vi "System2.vi"() -> ()   [LabVIEW 2013]
uses:
  <vilib>/imath/engines/lvmath/Functions/Error Handling/error.ctl
  <vilib>/imath/engines/lvmath/Plug In/_Char/NIMS_CH_character datatype.ctl
  <instrlib>/niUSRP/niUSRP Fetch Rx Data (CDB).vi
  <vilib>/imath/engines/lvmath2/RunTimeEngine/ErrorHandling/NIMS_Finalize Error.vi
  <vilib>/imath/engines/lvmath2/RunTimeEngine/Managers/WorkSpace/UID Generator.vi
  <vilib>/imath/engines/lvmath2/RunTimeEngine/NonStaticBuiltInFunctions/Manual/NIMS_NS_load.vi
  <vilib>/imath/engines/lvmath2/RunTimeEngine/RunTimeType/NIMS_RunTimeType_From StrictType (excl LVString).vi
  <instcachedir>/0/NIMS_RunTimeType_From StrictType (excl LVString)_4DEE718D6EB74582AA20236969C084FC.lvgen/NIMS_RunTimeType_From StrictType (excl LVString)_4DEE718D6EB74582AA20236969C084FC_000.vi
  <vilib>/imath/engines/lvmath2/RunTimeEngine/Managers/SymbolTable/Write Variable.vi
  <vilib>/imath/engines/lvmath2/RunTimeEngine/RowToken/NIMS_RowToken-nonstatic.vi
  <vilib>/imath/engines/lvmath2/RunTimeEngine/MatrixToken/NIMS_MatrixToken-nonstatic.vi
  <vilib>/imath/engines/lvmath2/RunTimeEngine/RunTimeSymbolToken/NIMS_RunTimeSymbolToken_ReadVariable-1out.vi
  <vilib>/imath/engines/lvmath/Functions/Error Handling/MergeErrorsWrapper.vi
  <vilib>/imath/engines/lvmath2/RunTimeEngine/LocalVariableDefStatement/MC_LocalVariableDefStatement_Display.vi
  <vilib>/imath/engines/lvmath2/RunTimeEngine/RunTimeSymbolToken/NIMS_RunTimeSymbolToken_ResolveSymbol.vi
  <instcachedir>/0/NIMS_RunTimeSymbolToken_ResolveSymbol_F94DACEDB8D84373A3303A9E667D843C.lvgen/NIMS_RunTimeSymbolToken_ResolveSymbol_F94DACEDB8D84373A3303A9E667D843C_003.vi
  <vilib>/imath/engines/lvmath2/RunTimeEngine/CommandStatement/NIMS_CommandStatement_MaskErr.vi
  <vilib>/imath/engines/lvmath2/RunTimeEngine/Managers/SymbolTable/Read Variable.vi
  <vilib>/imath/engines/lvmath2/RunTimeEngine/RunTimeType/NIMS_RunTimeType_Get Case Value.vi
  <vilib>/imath/engines/lvmath2/RunTimeEngine/NodeEndStatement/MC_NodeEndStatement_Dispose.vi
  <vilib>/imath/engines/lvmath2/RunTimeEngine/NodeEndStatement/NIMS_NodeEndStatement_Output.vi
  <instcachedir>/0/NIMS_NodeEndStatement_Output_53EC0D466D134D7ABD903AC30B43404B.lvgen/NIMS_NodeEndStatement_Output_53EC0D466D134D7ABD903AC30B43404B_004.vi
  <vilib>/imathl/engines/lvmath/Functions/Error Handling/Create Error.vi
  <vilib>/imath/engines/lvmath2/RunTimeEngine/RunTimeType/NIMS_RunTimeType_To Numeric.vi
  <instcachedir>/0/NIMS_RunTimeType_To Numeric_4795FB10E831402FABFA341B47E20681.lvgen/NIMS_RunTimeType_To Numeric_4795FB10E831402FABFA341B47E20681_000.vi
  <vilib>/imath/engines/lvmath2/RunTimeEngine/NodeEndStatement/NIMS_NodeEndStatement_Get Vector.vi
  <instcachedir>/0/NIMS_NodeEndStatement_Get Vector_BE4364D373AE46158CA0B14DEB6F98C8.lvgen/NIMS_NodeEndStatement_Get Vector_BE4364D373AE46158CA0B14DEB6F98C8_003.vi
  <vilib>/imath/engines/lvmath/Plug In/_Char/RunTimeType/NIMS_CH_RunTimeType_To Character 2D.vi
  <instcachedir>/0/NIMS_NodeEndStatement_Get Vector_BE4364D373AE46158CA0B14DEB6F98C8.lvgen/NIMS_NodeEndStatement_Get Vector_BE4364D373AE46158CA0B14DEB6F98C8_000.vi
  <vilib>/imath/engines/lvmath/Plug In/_Char/NIMS_CH_Character 1D to U8 1D.vi
  <vilib>/imath/engines/lvmath2/RunTimeEngine/BuiltInFunctions/crosscorr/NIMS_crosscorr(GV,GV,Str).vi
  <instcachedir>/0/NIMS_crosscorr(GV,GV,Str)_7F516622EB1B4986A7D0F3F178AC2F2E.lvgen/NIMS_crosscorr(GV,GV,Str)_7F516622EB1B4986A7D0F3F178AC2F2E_000.vi
  <vilib>/imath/engines/lvmath2/RunTimeEngine/BuiltInFunctions/abs/NIMS_abs(signed).vi
  <instcachedir>/0/NIMS_abs(signed)_C4FCB8E6058B49B797C7C8D53CA5F6EC.lvgen/NIMS_abs(signed)_C4FCB8E6058B49B797C7C8D53CA5F6EC_006.vi
  <vilib>/imath/engines/lvmath2/RunTimeEngine/BuiltInFunctions/length/NIMS_length(GV).vi
  <instcachedir>/0/NIMS_length(GV)_08A3D13377FD4E4B96F5795FBF3698FA.lvgen/NIMS_length(GV)_08A3D13377FD4E4B96F5795FBF3698FA_001.vi
  <vilib>/imath/engines/lvmath2/RunTimeEngine/RangeToken/NIMS_Range_R2 - Integer.vi
  <instcachedir>/0/NIMS_Range_R2 - Integer_C51C130E5EA5464EA148B28CDAB9615A.lvgen/NIMS_Range_R2 - Integer_C51C130E5EA5464EA148B28CDAB9615A_000.vi
  <instcachedir>/0/NIMS_NodeEndStatement_Output_53EC0D466D134D7ABD903AC30B43404B.lvgen/NIMS_NodeEndStatement_Output_53EC0D466D134D7ABD903AC30B43404B_014.vi
  <instcachedir>/0/NIMS_NodeEndStatement_Output_53EC0D466D134D7ABD903AC30B43404B.lvgen/NIMS_NodeEndStatement_Output_53EC0D466D134D7ABD903AC30B43404B_011.vi
  <vilib>/imath/engines/lvmath2/RunTimeEngine/IndexRead/NIMS V(S).vi
  <instcachedir>/0/NIMS V(S)_0488751826AF41519A22953C041130DC.lvgen/NIMS V(S)_0488751826AF41519A22953C041130DC_005.vi
  <instcachedir>/0/NIMS_abs(signed)_C4FCB8E6058B49B797C7C8D53CA5F6EC.lvgen/NIMS_abs(signed)_C4FCB8E6058B49B797C7C8D53CA5F6EC_002.vi
  <vilib>/imath/engines/lvmath2/RunTimeEngine/ErrorHandling/NIMS_Create Error From Enums.vi
  <vilib>/imath/engines/lvmath2/RunTimeEngine/Managers/SymbolTable/Clear UID.vi
  <vilib>/imath/engines/lvmath2/RunTimeEngine/BuiltInFunctions/close/NIMS_close(Enums).vi
  <vilib>/imath/engines/lvmath2/RunTimeEngine/BuiltInFunctions/figure/NIMS_figure(I32).vi
  <vilib>/imath/engines/lvmath2/RunTimeEngine/BuiltInFunctions/plot/NIMS_plot(G, Str).vi
  <instcachedir>/0/NIMS_plot(G, Str)_30D49D8623E0484DBD39D394DDFCBE95.lvgen/NIMS_plot(G, Str)_30D49D8623E0484DBD39D394DDFCBE95_000.vi
  <instcachedir>/0/NIMS_NodeEndStatement_Output_53EC0D466D134D7ABD903AC30B43404B.lvgen/NIMS_NodeEndStatement_Output_53EC0D466D134D7ABD903AC30B43404B_000.vi
  <instcachedir>/0/NIMS_NodeEndStatement_Output_53EC0D466D134D7ABD903AC30B43404B.lvgen/NIMS_NodeEndStatement_Output_53EC0D466D134D7ABD903AC30B43404B_001.vi
  <vilib>/imath/engines/lvmath/Plug In/_Char/NIMS_CH_Character RV to String.vi
  <instcachedir>/0/NIMS_plot(G, Str)_30D49D8623E0484DBD39D394DDFCBE95.lvgen/NIMS_plot(G, Str)_30D49D8623E0484DBD39D394DDFCBE95_001.vi
  <vilib>/imath/engines/lvmath2/RunTimeEngine/BuiltInFunctions/hold/NIMS_hold(Enums).vi
  <vilib>/imath/engines/lvmath2/RunTimeEngine/IndexRead/NIMS V(R2).vi
  <instcachedir>/0/NIMS V(R2)_C76619605A0E4E9F8B2FA9389712AC47.lvgen/NIMS V(R2)_C76619605A0E4E9F8B2FA9389712AC47_001.vi
  <vilib>/imath/engines/lvmath2/RunTimeEngine/BuiltInFunctions/max/1 input/NIMS_max(RV).vi
  <instcachedir>/0/NIMS_max(RV)_237633DB1D604D5BA7001287DF3C7957.lvgen/NIMS_max(RV)_237633DB1D604D5BA7001287DF3C7957_000.vi
  <instcachedir>/0/NIMS_length(GV)_08A3D13377FD4E4B96F5795FBF3698FA.lvgen/NIMS_length(GV)_08A3D13377FD4E4B96F5795FBF3698FA_002.vi
  <vilib>/imath/engines/lvmath2/RunTimeEngine/BuiltInFunctions/angle/NIMS_angle.vi
  <instcachedir>/0/NIMS_angle_6DDAE2BD99E0421EB990B6436E94D88F.lvgen/NIMS_angle_6DDAE2BD99E0421EB990B6436E94D88F_005.vi
  <vilib>/imath/engines/lvmath2/RunTimeEngine/BuiltInFunctions/imag/NIMS_imag(Complex).vi
  <instcachedir>/0/NIMS_imag(Complex)_3180D40D00C843A49C2B33397F857BF3.lvgen/NIMS_imag(Complex)_3180D40D00C843A49C2B33397F857BF3_002.vi
  <vilib>/imath/engines/lvmath2/RunTimeEngine/RangeToken/NIMS_Range.vi
  <instcachedir>/0/NIMS_Range_7481B155BEE341ECA0F59DDB444E2C09.lvgen/NIMS_Range_7481B155BEE341ECA0F59DDB444E2C09_001.vi
  <vilib>/imath/engines/lvmath2/RunTimeEngine/IndexRead/NIMS V(V).vi
  <instcachedir>/0/NIMS V(V)_298D9CB7BFEB42B8BC8D9C3C28AE8C70.lvgen/NIMS V(V)_298D9CB7BFEB42B8BC8D9C3C28AE8C70_000.vi
  <vilib>/imath/engines/lvmath2/RunTimeEngine/BuiltInFunctions/mean/NIMS_CS=mean(CV,I32).vi
  <instcachedir>/0/NIMS_angle_6DDAE2BD99E0421EB990B6436E94D88F.lvgen/NIMS_angle_6DDAE2BD99E0421EB990B6436E94D88F_003.vi
  <vilib>/imath/engines/lvmath2/RunTimeEngine/BuiltInFunctions/mean/NIMS_RS=mean(RV,I32).vi
  <instcachedir>/0/NIMS_abs(signed)_C4FCB8E6058B49B797C7C8D53CA5F6EC.lvgen/NIMS_abs(signed)_C4FCB8E6058B49B797C7C8D53CA5F6EC_000.vi
  <vilib>/imath/engines/lvmath2/RunTimeEngine/BuiltInFunctions/linramp/NIMS_linramp.vi
  <vilib>/imath/engines/lvmath2/RunTimeEngine/ArithmeticOperatorToken/NIMS_ArithmeticOperator_plus.vi
  <instcachedir>/0/NIMS_ArithmeticOperator_plus_8A46DAFC24D445C9B2C97B626139369E.lvgen/NIMS_ArithmeticOperator_plus_8A46DAFC24D445C9B2C97B626139369E_005.vi
  <vilib>/imath/engines/lvmath2/RunTimeEngine/BuiltInFunctions/numelements/NIMS_numelements.vi
  <instcachedir>/0/NIMS_numelements_A776DA77F73142F68C2F209B523114C5.lvgen/NIMS_numelements_A776DA77F73142F68C2F209B523114C5_003.vi
  <vilib>/imath/engines/lvmath2/RunTimeEngine/BuiltInFunctions/zeros/NIMS_V=zeros(I32,I32).vi
  <vilib>/imath/engines/lvmath2/RunTimeEngine/CommandStatement/MC_CommandStatement_break.vi
  LabVIEW Data/MathScriptVIs/MCStatic_31879994332_13cee6d0e2951097849577d15734aa47.vi
  <instcachedir>/0/MCStatic_31879994332_13cee6d0e2951097849577d15734aa47_76F944008E9241CE9E75835197D7770E.lvgen/MCStatic_31879994332_13cee6d0e2951097849577d15734aa47_76F944008E9241CE9E75835197D7770E_000.vi
  <vilib>/imath/engines/lvmath2/RunTimeEngine/IndexReplace/NIMS V(S)=S.vi
  <instcachedir>/0/NIMS V(S)=S_66A18068148B4981A312229A93EA5C06.lvgen/NIMS V(S)=S_66A18068148B4981A312229A93EA5C06_001.vi
  <instcachedir>/0/NIMS V(S)=S_66A18068148B4981A312229A93EA5C06.lvgen/NIMS V(S)=S_66A18068148B4981A312229A93EA5C06_000.vi
  <vilib>/imath/engines/lvmath2/RunTimeEngine/BuiltInFunctions/round/NIMS_round(DBL-S).vi
  <vilib>/imath/engines/lvmath2/RunTimeEngine/BuiltInFunctions/title/NIMS_title.vi
  <instcachedir>/0/NIMS V(S)_0488751826AF41519A22953C041130DC.lvgen/NIMS V(S)_0488751826AF41519A22953C041130DC_000.vi
  <vilib>/imath/engines/lvmath2/RunTimeEngine/BuiltInFunctions/grid/NIMS_grid(Enums).vi
  <instcachedir>/0/NIMS_abs(signed)_C4FCB8E6058B49B797C7C8D53CA5F6EC.lvgen/NIMS_abs(signed)_C4FCB8E6058B49B797C7C8D53CA5F6EC_001.vi
  <vilib>/imath/engines/lvmath2/RunTimeEngine/BuiltInFunctions/min/1 input/NIMS_min(RV).vi
  <instcachedir>/0/NIMS_min(RV)_EE2DD3E2888846108C5160A664B67832.lvgen/NIMS_min(RV)_EE2DD3E2888846108C5160A664B67832_000.vi
  <vilib>/imath/engines/lvmath2/RunTimeEngine/IndexRead/NIMS M(S,S).vi
  <instcachedir>/0/NIMS M(S,S)_AC51E74150A542F7991B9634C66F3096.lvgen/NIMS M(S,S)_AC51E74150A542F7991B9634C66F3096_003.vi
  <vilib>/imath/engines/lvmath2/RunTimeEngine/IndexRead/NIMS M(S,$).vi
  <instcachedir>/0/NIMS M(S,$)_F24F360562DE41D8BE234322A2E15C65.lvgen/NIMS M(S,$)_F24F360562DE41D8BE234322A2E15C65_002.vi
  <vilib>/imath/engines/lvmath2/RunTimeEngine/BuiltInFunctions/min/2 inputs/NIMS_min(RG,RG)-no size check.vi
  <instcachedir>/0/NIMS_min(RG,RG)-no size check_7F67BAB91AFC452D9517D2EA1C8F5F88.lvgen/NIMS_min(RG,RG)-no size check_7F67BAB91AFC452D9517D2EA1C8F5F88_001.vi
  <instcachedir>/0/NIMS V(R2)_C76619605A0E4E9F8B2FA9389712AC47.lvgen/NIMS V(R2)_C76619605A0E4E9F8B2FA9389712AC47_002.vi
  <vilib>/imath/engines/lvmath2/RunTimeEngine/ArithmeticOperatorToken/NIMS_ArithmeticOperator_minus.vi
  <instcachedir>/0/NIMS_ArithmeticOperator_minus_5462A7974F41415E96B34B7C9D041F4F.lvgen/NIMS_ArithmeticOperator_minus_5462A7974F41415E96B34B7C9D041F4F_016.vi
  <instcachedir>/0/NIMS_abs(signed)_C4FCB8E6058B49B797C7C8D53CA5F6EC.lvgen/NIMS_abs(signed)_C4FCB8E6058B49B797C7C8D53CA5F6EC_007.vi
  <vilib>/imath/engines/lvmath2/RunTimeEngine/BuiltInFunctions/sum/NIMS_sum(GV).vi
  <instcachedir>/0/NIMS_sum(GV)_67F5EC36BC034E54A6BEC5B0673C00E5.lvgen/NIMS_sum(GV)_67F5EC36BC034E54A6BEC5B0673C00E5_000.vi
  <instcachedir>/0/NIMS_crosscorr(GV,GV,Str)_7F516622EB1B4986A7D0F3F178AC2F2E.lvgen/NIMS_crosscorr(GV,GV,Str)_7F516622EB1B4986A7D0F3F178AC2F2E_001.vi
  MATLAB_func/frequency_synchronisation_sample.m
  <vilib>/imath/engines/lvmath2/RunTimeEngine/Managers/SymbolTable/NIMS_WorkSpace.lvlib
panel:
  out "error":dbl
  out "size(s)":i32
  out "length_signal_out":i32
  in  "file (use dialog) 2":path
  in  "file (use dialog)":path
  out "time":dbl
  out "a":cdb[](array[numeric])
  in  "message number of samples (50000)":i64=100000
  out "index":i32
  in  "stop 2":bool
  in  "Wakeup #samples (100)":i64=100000
  out "RX coerced gain":dbl format="%#_6f"
  out "RX coerced IQ rate":dbl=100000.0 format="%#_6p"
  in  "RX gain":dbl format="%#_6f"
  in  "RX IQ rate":dbl=100000.0 format="%#_6p"
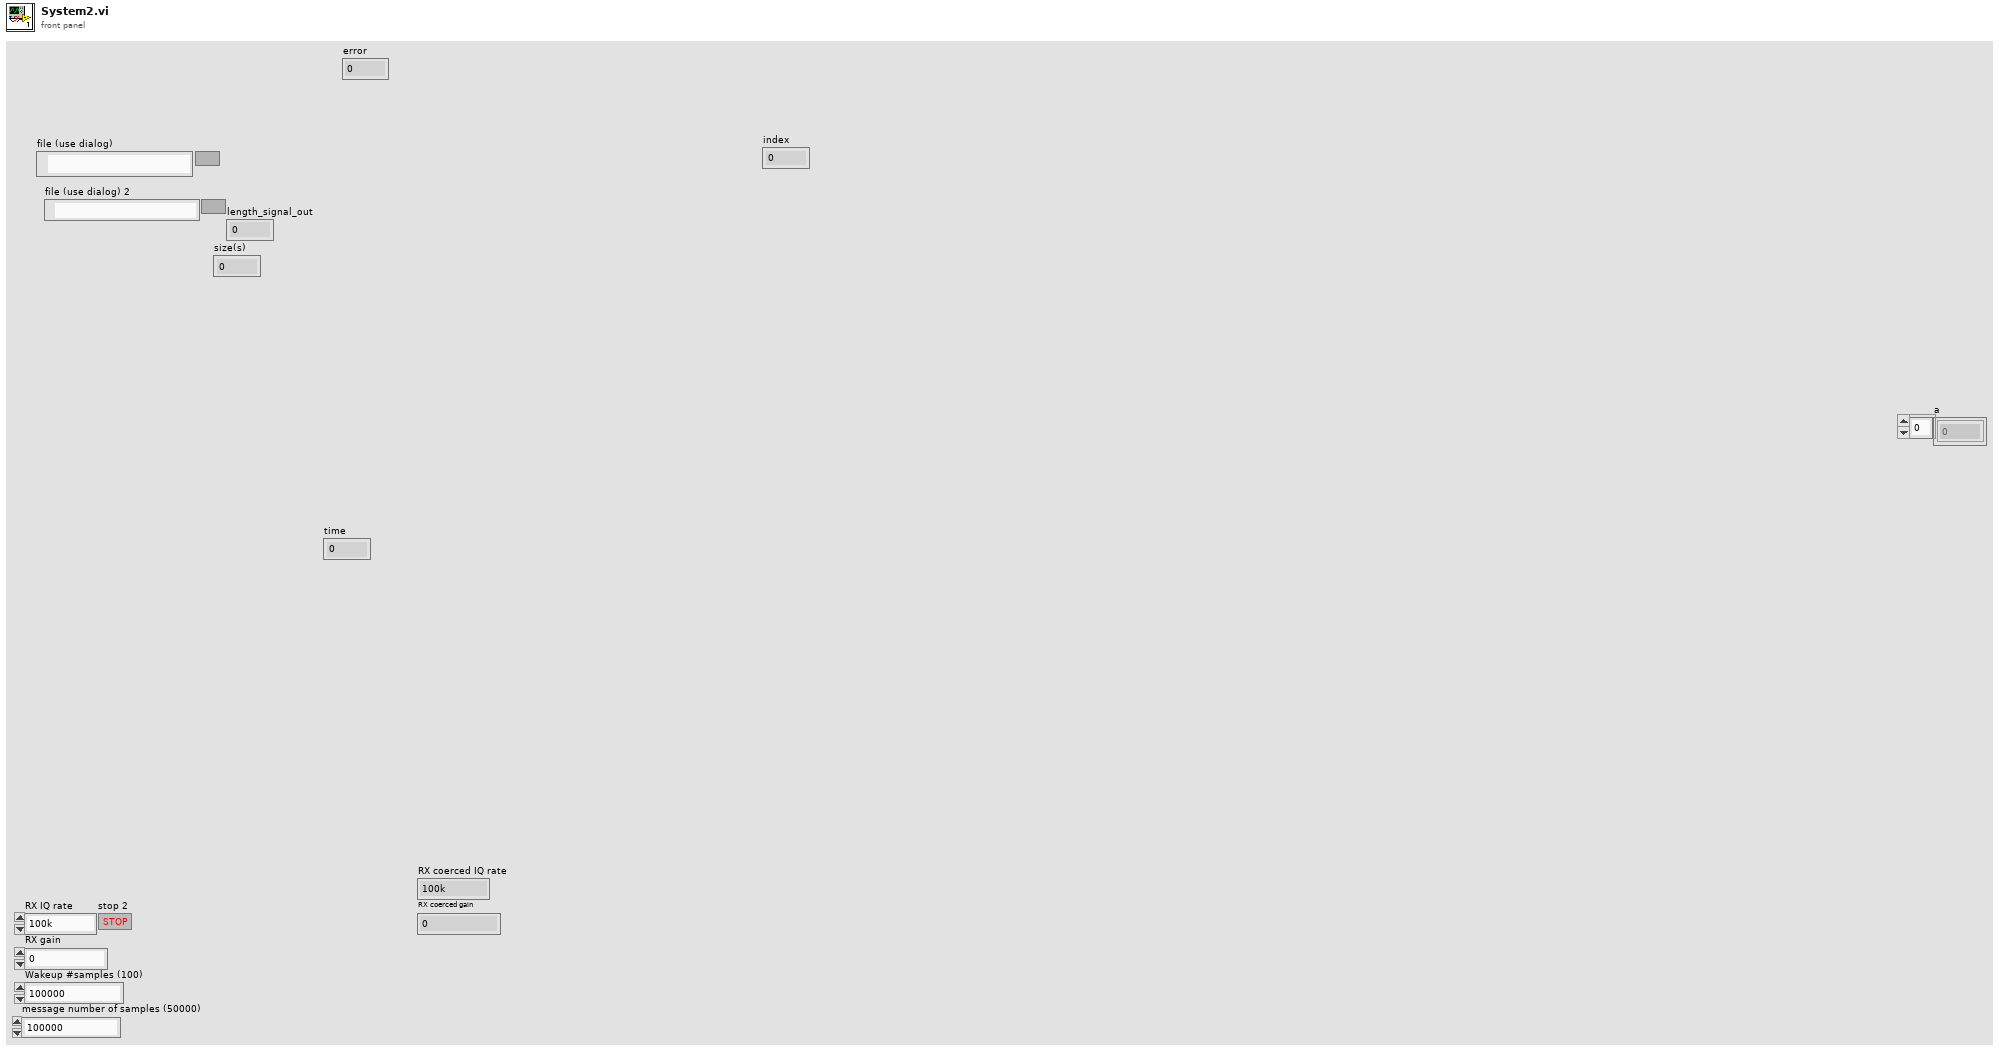
[diagram p1: front panel]
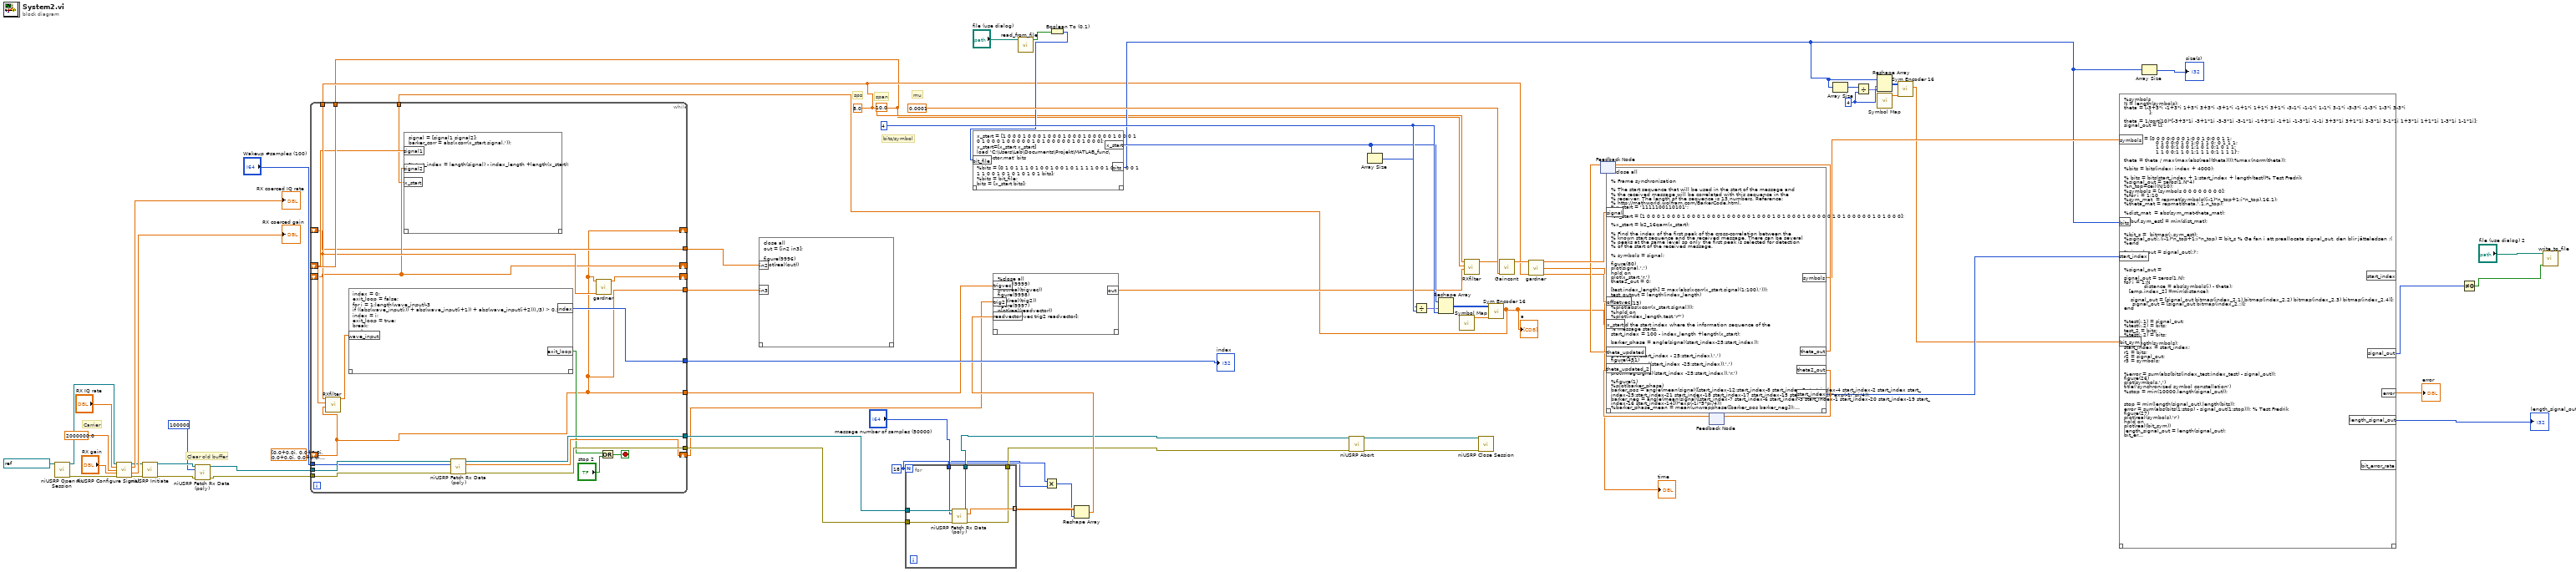
[diagram p0: block diagram]
diagram:
  w14 = 4 ("dimension size")
  w26 = 18
  w8 = 8.0 ("span")
  w55 = 4 ("dimension size")
  w7 = 10.0 ("span")
  # "Clear old buffer"
  # "sps"
  # "bits/symbol"
  # "span"
  # "mu"
  # "Carrier"
  n1 = call <instrlib>:"niUSRP Open Rx Session.vi"("device names"=refnum<k15> "192.168.10.9") -> ("session handle out"=w70:refnum<k15>, "error out"=w68:errorcluster)  [unwired: 13 in]
  n2 = call <instrlib>:"niUSRP Configure Signal.vi"("session handle"=w70, "IQ rate"="RX IQ rate", "carrier frequency"=2000000.0, "gain"="RX gain", "error in (no error)"=w68) -> ("session handle out"=w61:refnum<k15>, "coerced IQ rate"=→"RX coerced IQ rate":dbl, "coerced gain"=→"RX coerced gain":dbl, "error out"=w60:errorcluster)  [unwired: 6 in, 1 out]
  n3 = call <instrlib>:"niUSRP Initiate.vi"("session handle"=w61, "error in (no error)"=w60) -> ("session handle out"=w36:refnum<k15>, "error out"=w37:errorcluster)  [unwired: 12 in]
  n4 = call-poly <instrlib>:"niUSRP Fetch Rx Data (poly).vi"("session handle"=w36, "number of samples"=i64 100000, "error in (no error)"=w37) -> ("session handle out"=w39:refnum<k15>, "error out"=w38:errorcluster)  [unwired: 9 in, 2 out]
  n5 = call "read_from_file.vi"("file (use dialog)"="file (use dialog)") -> ("data"=w23:bool[])  [unwired: 10 in]
  n6 = Multiply(x="message number of samples (50000)", y=w26) -> (x*y=w28:i64)
  n7 = Boolean To (0,1)(Boolean=w23) -> (0, 1=w22:i16[])
  n8 = mathscript code="x_start = [1 0 0 0 1 0 0 0 1 0 0 0 1 0 0 0 1 0 0 0 0 0 1 0 0 0 1 0 1 0 0 0 1 0 0 0 0 0 1 0 1 0 0 0 0 0 1 0 1 0 0 0];\nx_start=[x_start x_start]\nload 'C:\\Users\\Lab\\Documents\\Projekt\\MATLAB_func\\testvector.mat' bits\n\n%bits = [0 1 0 1 1 1 0 1 0 0 1 0 0 1 0 1 1 1 1 0 0 1 0 1 0 0 0 1 1 1 0 0 1 0 1 0 1 0 1 0 1 bits];\n%bits = bit_file;\nbits = [x_start bits];"("bit_file"=w22) -> ("x_start"=w48:i32[], "bits"=w11:i32[])  [unwired: 1 in, 1 out]
  n9 = Array Size(array=w48) -> (size(s)=w49:i32)
  n10 = Divide(x=w49, y=w55) -> (x/y=w54:fxp<+,27,27>)
  n11 = Reshape Array(w48, w54, w55) -> (w52:i32[][])
  n12 = call "Symbol Map.vi"() -> ("symbol_map"=w56:cdb[])  [unwired: 11 in]
  n13 = call "Sym Encoder 16.vi"("symbol_map"=w56, "b"=w52) -> ("a"=w6:cdb[])  [unwired: 9 in]
  "a" <- w6
  n14 = while {
    tunnel: w39 -> [w90]
    tunnel: w38 -> [w89]
    tunnel: [w88] -> w34
    tunnel: [w87] -> w33
    tunnel: "Wakeup #samples (100)" -> [w86]
    shift-right: [w85] -> w4
    shift-left: cdb[] [0.0+0.0i, 0.0+0.0i, 0.0+0.0i, 0.0+0.0i, 0.0+0.0i, 0.0+0.0i, 0.0+0.0i, 0.0+0.0i, 0.0+0.0i, 0.0+0.0i, 0.0+0.0i, 0.0+0.0i, 0.0+0.0i, 0.0+0.0i, 0.0+0.0i, 0.0+0.0i, 0.0+0.0i] ("data") -> [w73]
    tunnel: [w84] -> w58
    tunnel: [w73] -> w5
    tunnel: w8 -> [w78]
    tunnel: w7 -> [w80]
    shift-right: [w79] -> _
    shift-left: _ -> [w76]
    shift-right: [w76] -> _
    shift-left: _ -> [w77]
    tunnel: w6 -> [w75]
    tunnel: [w73] -> w3
    tunnel: [w74] -> w1
    shift-right: [w73] -> _
    shift-left: _ -> [w74]
    stop <- w82 stop-if-true
    n15 = call "RXfilter.vi"("Array"=w73, "span"=w80, "sps"=w78) -> ("out"=w72:cdb[])  [unwired: 8 in]
    n16 = mathscript code="index = 0;\nexit_loop = false;\nfor i = 1:length(wave_input)-3\nif ((abs(wave_input(i)) + abs(wave_input(i+1)) + abs(wave_input(i+2)))./3) > 0.5\nindex = i;\nexit_loop = true;\nbreak;\nend\nend"("wave_input"=w72) -> ("index"=w84:i32, "exit_loop"=w81:bool)  [unwired: 1 in, 1 out]
    n17 = mathscript code="signal = [signal1 signal2];\nbarker_corr = abs(xcorr(x_start,signal.'));\n\n\n\n%start_index = length(signal) - index_length +length(x_start);"("signal1"=w77, "signal2"=w76, "x_start"=w75) -> ()  [unwired: 1 in, 1 out]
    n18 = call-poly <instrlib>:"niUSRP Fetch Rx Data (poly).vi"("session handle"=w90, "number of samples"=w86, "error in (no error)"=w89) -> ("session handle out"=w88:refnum<k15>, "data"=w85:cdb[], "error out"=w87:errorcluster)  [unwired: 9 in, 1 out]
    n19 = call "gardner.vi"("in"=w73, "sps"=w78) -> ("sym"=w79:cdb[])  [unwired: 11 in, 2 out]
    n20 = Or(x=w81, y="stop 2") -> (x .or. y?=w82:bool)
  }
  "index" <- w58
  n21 = mathscript code="close all\nout = [in2 in3];\n\nfigure(9996)\nplot(real(out))"("in2"=w1, "in3"=w3) -> ()  [unwired: 1 in, 1 out]
  n22 = for {
    N: w26 -> [_]
    tunnel: w34 -> [w265]
    tunnel: w33 -> [w264]
    tunnel: [w263] -> w32 mode=indexing
    tunnel: "message number of samples (50000)" -> [w262]
    tunnel: [w261] -> w30
    tunnel: [w260] -> w29
    n23 = call-poly <instrlib>:"niUSRP Fetch Rx Data (poly).vi"("session handle"=w265, "number of samples"=w262, "error in (no error)"=w264) -> ("session handle out"=w261:refnum<k15>, "data"=w263:cdb[], "error out"=w260:errorcluster)  [unwired: 9 in, 1 out]
  }
  n24 = Reshape Array(w32, w28) -> (w31:cdb[])
  n25 = mathscript code="%close all\nfigure(9999)\nplot(real(trigvec))\nfigure(9998)\nplot(real(trig2))\nfigure(9997)\nplot(real(readvector))\nout = [trigvec trig2 readvector];"("trigvec"=w5, "trig2"=w4, "readvector"=w31) -> ("out"=w50:cdb[])  [unwired: 1 in, 1 out]
  n26 = call <instrlib>:"niUSRP Abort.vi"("session handle"=w30, "error in (no error)"=w29) -> ("session handle out"=w69:refnum<k15>, "error out"=w67:errorcluster)  [unwired: 12 in]
  n27 = call "RXfilter.vi"("Array"=w50, "span"=w7, "sps"=w8) -> ("out"=w51:cdb[])  [unwired: 8 in]
  n28 = call <instrlib>:"niUSRP Close Session.vi"("session handle"=w69, "error in (no error)"=w67) -> ()  [unwired: 13 in, 1 out]
  n29 = call "Gaincont.vi"("mu"=0.0001, "Array"=w51) -> ("out"=w53:cdb[])  [unwired: 9 in]
  n30 = call "gardner.vi"("in"=w53, "sps"=w8) -> ("sym"=w47:cdb[], "time"=→"time":dbl, "offsetvec"=w40:dbl[])  [unwired: 11 in]
  n31 = feedback #1() -> (w43:dbl)  [unwired: 1 in]
  n32 = feedback #2() -> (w45:dbl)  [unwired: 1 in]
  n33 = mathscript code="%close all\n\n% Frame synchronisation\n\n% The start sequence that will be used in the start of the message and\n% the received message will be correlated with this sequence in the \n% receiver. The length of the sequence is 13 numbers. Reference: \n% http://mathworld.wolfram.com/BarkerCode.html.\n%x_start = '1111100110101';\n\n%x_start = [1 0 0 0 1 0 0 0 1 0 0 0 1 0 0 0 1 0 0 0 0 0 1 0 0 0 1 0 1 0 0 0 1 0 0 0 0 0 1 0 1 0 0 0 0 0 1 0 1 0 0 0];\n\n%x_start = b2_16qam(x_start);\n\n% Find the index of the first peak of the cross-correlation between the \n% known start sequence and the received message. There can be several \n% peaks at the same level so only the first peak is selected for detection \n% of the start of the received message.\n\n% symbols = signal;\n\nfigure(80)\nplot(signal,'.')\nhold on\nplot(x_start,'r.')\ntheta2_out = 0;\n\n[test,index_length] = max(abs(xcorr(x_start,signal(1:100).')));\ntest_output = length(index_length)\n\n%figure(13)\n%plot(abs(xcorr(x_start,signal)));\n%hold on\n%plot(index_length,test,'r*')\n\n% Find the start index where the information sequence of the \n% message starts.\nstart_index = 100 - index_length +length(x_start);\n\nbarker_phase = angle(signal(start_index-25:start_index));\n\nfigure(450)\nplot(signal(start_index - 25:start_index),'.')\nfigure(451)\nplot(real(signal(start_index -25:start_index)),'.')\nhold on\nplot(imag(signal(start_index -25:start_index)),'r.')\n\n%figure(1)\n%plot(barker_phase)\nbarker_pos = angle(mean(signal([start_index-12:start_index-8 start_index-5 start_index-4 start_index-2 start_index start_index-25:start_index-21 start_index-18 start_index-17 start_index-15 start_index-13]))*exp(-1i*pi/4)); \nbarker_neg = angle(mean(signal([start_index-7 start_index-6 start_index-3 start_index-1 start_index-20 start_index-19 start_index-16 start_index-14]))*exp(-1i*5*pi/4)); \n%barker_phase_mean = mean(unwrapphase([barker_pos barker_neg]));\n\nbarker_phase_mean = -mean([mean(barker_pos) mean(barker_neg)]);\nif (abs(mean((barker_pos))-mean((barker_neg)))>pi)\nbarker_phase_mean=barker_phase_mean+pi;\nend;\nphi_updated = barker_phase_mean;\n\nexact_value =1.2; %(abs(3 + 1i.*3) + abs(3 + 1i.*1))./2;\nrad = linspace(0,2*pi,1000);\ncircle = exact_value*(cos(rad)+1i*sin(rad));\n%signal = signal/(1.25/0.8);\nfigure(17)\nplot(signal,'.')\nhold on\nplot(circle,'r')\n\nN=numel(signal);\nsignal_corrected=zeros(1,N);\ntheta_updated_2_vec = zeros(1,N);\ntheta_updated_vec = zeros(1,N);\nphi_updated_vec = zeros(1,N);\n\nfor ind= 4:N\n % if (abs(signal(ind)) > exact_value && abs(signal(ind - 1)) > exact_value && ...\n   %        abs(signal(ind - 2)) > exact_value && ...\n    %       abs(signal(ind - 3)) > exact_value && first_start == 1 && running==0)\n      % [signal_corrected(ind - 3),phi_updated] = ...\n       %    phase_synchronisation_sample(signal(ind - 3),phi_updated,1);\n%      running=1;\n   % else\n        [signal_corrected(ind - 3),phi_updated,theta_updated,...\n            theta_updated_2] = frequency_synchronisation_sample(...\n            signal(ind-3),phi_updated,theta_updated,theta_updated_2,exact_value);\n%    end\n    theta_updated_2_vec(ind-3) = theta_updated_2;\n    theta_updated_vec(ind-3) = theta_updated;\n    phi_updated_vec(ind-3) = phi_updated;\n    if (ind == N)\n        for a = 1:3\n            [signal_corrected(N - 3 + a),phi_updated,theta_updated,theta_updated_2] = ...\n                frequency_synchronisation_sample(signal(N - 3 + a),...\n                phi_updated,theta_updated,theta_updated_2,exact_value);\n        end\n    end\n\nend\nfigure(28)\nplot(signal_corrected(1:end),'.')\ntest_rotation = angle(signal_corrected(1));\nfigure(452)\nplot(real(signal_corrected(start_index -25:start_index)),'.')\nhold on\nplot(imag(signal_corrected(start_index -25:start_index)),'r.')\n%barker_pos = angle(signal_corrected([start_index-12:start_index-8 start_index-5 start_index-4 start_index-2 start_index])*exp(-1i*pi/4)); \n%barker_neg = angle(signal_corrected([start_index-7 start_index-6 start_index-3 start_index-1])*exp(-1i*5*pi/4)); \nbarker_pos = angle(mean(signal_corrected([start_index-12:start_index-8 start_index-5 start_index-4 start_index-2 start_index start_index-25:start_index-21 start_index-18 start_index-17 start_index-15 start_index-13]))*exp(-1i*pi/4)); \nbarker_neg = angle(mean(signal_corrected([start_index-7 start_index-6 start_index-3 start_index-1 start_index-20 start_index-19 start_index-16 start_index-14]))*exp(-1i*5*pi/4)); \n%barker_phase_mean = mean(unwrapphase([barker_pos barker_neg]));\n%barker_pos=unwrapphase(barker_pos)\n%barker_neg=unwrapphase(barker_neg)\nbarker_phase_mean = -mean([mean(barker_pos) mean(barker_neg)]);\nif (abs(mean((barker_pos))-mean((barker_neg)))>pi)\nbarker_phase_mean=barker_phase_mean+pi;\nend\ntest_phase = barker_phase_mean;\n\n% barker_phase_mean = mean(unwrapphase(barker_pos));\nphi_updated_2 = barker_phase_mean;\nphi_updated_2 =round(phi_updated_2./(pi/2))*pi/2;\n\n\n\n\nfigure(400)\nplot(real(signal_corrected))\n\n% Test Fredrik and Fredrik\n% symbols = signal_corrected(start_index + 1:start_index + 5000).*exp(1i*phi_updated_2);\nstop = length(signal_corrected(start_index + 1:end));\n\nsymbols = signal_corrected(1:stop).*exp(1i*phi_updated_2);\n\n\nfigure(455)\ntitle('Barker sequence after synchronisation.')\nplot(real(symbols(start_index -25:start_index)),'.')\nhold on\nplot(imag(symbols(start_index -25:start_index)),'r.')\n\nsymbols = symbols(start_index  - 25:end);\n%symbols = signal_corrected;\n\nfigure(401)\nplot(real(symbols))\n\nphi_out=phi_updated_vec(N-4);\ntheta_out=theta_updated_vec(N-5);\ntheta2_out=theta_updated_2_vec(N-4);\nfigure(8888)\nplot(theta_updated_2_vec)\ntitle('Accumulated frequency phase correction');\nfigure(479)\nplot(phi_updated_vec)\ntitle('Phase offset per symbol');\nhold off\nfigure(1337)\nplot(symbols(1:end-1),'.')\ngrid on"("x_start"=w6, "signal"=w47, "theta_updated_2"=w45, "theta_updated"=w43, "offsetvec"=w40) -> ("theta2_out"=w46:dbl, "theta_out"=w44:dbl, "start_index"=w42:i32, "symbols"=w41:cdb[])  [unwired: 1 in, 1 out]
  n34 = feedback-in #1(w44) -> ()
  n35 = feedback-in #2(w46) -> ()
  n36 = Array Size(array=w11) -> (size(s)=w12:i32)
  n37 = Divide(x=w12, y=w14) -> (x/y=w13:fxp<+,27,27>)
  n38 = Reshape Array(w11, w13, w14) -> (w15:i32[][])
  n39 = call "Symbol Map.vi"() -> ("symbol_map"=w16:cdb[])  [unwired: 11 in]
  n40 = call "Sym Encoder 16.vi"("symbol_map"=w16, "b"=w15) -> ("a"=w10:cdb[])  [unwired: 9 in]
  n41 = mathscript code="%symbols\nN = length(symbols);\ntheta = [-3+3*i -1+3*i 1+3*i 3+3*i -3+1*i -1+1*i 1+1*i 3+1*i -3-1*i -1-1*i 1-1*i 3-1*i -3-3*i -1-3*i 1-3*i 3-3*i\n               ];\n\ntheta = 1/sqrt(10)*[-3+3*1i -3+1*1i -3-3*1i -3-1*1i -1+3*1i -1+1i -1-3*1i -1-1i 3+3*1i 3+1*1i 3-3*1i 3-1*1i 1+3*1i 1+1*1i 1-3*1i 1-1*1i];\nsignal_out = [];\n\n\nbitmap = [0 0 0 0;0 0 0 1;0 0 1 0;0 0 1 1;\n                   0 1 0 0;0 1 0 1;0 1 1 0; 0 1 1 1;\n                   1 0 0 0;1 0 0 1;1 0 1 0;1 0 1 1;\n                   1 1 0 0;1 1 0 1;1 1 1 0;1 1 1 1]';\n\ntheta = theta / max(max(abs(real(theta))));%max(norm(theta));\n\n%bits = bits(index: index + 4000);\n\n% bits = bits(start_index + 1:start_index + length(test))% Test Fredrik\n%signal_out = zeros(1,N*4)\n%n_top=ceil(N/10);\n%symbols = [symbols 0 0 0 0 0 0 0 0];\n%for i = 1:10\n%sym_mat  = repmat(symbols((i-1)*n_top+1:i*n_top),16,1);\n%theta_mat = repmat(theta.',1,n_top);\n\n%dist_mat  = abs(sym_mat-theta_mat);\n\n%[buf,sym_est] = min(dist_mat);\n\n\n%bit_s =  bitmap(:,sym_est);\n%signal_out(:,(i-1)*n_top+1:i*n_top) = bit_s % Ge fan i att preallocata signal_out, den blir jätteledsen :(\n%end\n\n%signal_out = signal_out(:)';\n\n\n\n%signal_out = \n\nsignal_out = zeros(1,N);\nfor i = 1:N\n            distance = abs(symbols(i) - theta);\n   [emp,index_2] =min(distance);\n    \n    signal_out = [signal_out bitmap(index_2,1) bitmap(index_2,2) bitmap(index_2,3) bitmap(index_2,4)];\n     signal_out = [signal_out bitmap(index_2,:)];\nend\n\n\n%test(:,1) = signal_out;\n%test(:,2) = bits;\ntest_2 = bits;\n%test(:,2) = bits;\n\nN = length(symbols);\nstart_index = start_index;\nr1 = bits;\nr2 = signal_out;\nr3 = symbols;\n\n\n%error = sum(abs(bits(index_test:index_test) - signal_out));\nfigure(26)\nplot(symbols,'.')\ntitle('synchronized symbol constellation')\n%stop = min(10000,length(signal_out));\n\n\nstop = min(length(signal_out),length(bits));\nerror = sum(abs(bits(1:stop) - signal_out(1:stop))); % Test Fredrik\nfigure(27)\nplot(real(symbols),'r')\nhold on\nplot(real(bit_sym))\nlength_signal_out = length(signal_out);\nbit_error_rate = error./stop;\n\nfigure(350)\nplot(xcorr(error,bits(1:20000)))\n\n\nfigure(95)\nplot(symbols(50:end))\ntitle('test result')\n\nfigure(951)\nplot(symbols(1000:end),'.')"("start_index"=w42, "bits"=w11, "symbols"=w41, "bit_sym"=w10) -> ("length_signal_out"=→"length_signal_out":i32, "signal_out"=w21:i32[], "error"=→"error":dbl)  [unwired: 1 in, 3 out]
  n42 = Array Size(array=w11) -> (size(s)=→"size(s)":i32)
  n43 = Not Equal To 0?(x=w21) -> (x != 0?=w19:bool[])
  n44 = call "write_to_file.vi"("data 3"=w19, "file (use dialog) in"="file (use dialog) 2") -> ()  [unwired: 10 in]
